vi "testParseCommentsTrailingSlashSlash.vi"(8 "error in (no error)":errorcluster, 11 "testStateMachineUtilities in":refnum<class "testStateMachineUtilities.lvclass">) -> (0 "error out":errorcluster, 3 "testStateMachineUtilities out":refnum<class "testStateMachineUtilities.lvclass">)   [LabVIEW 2020, in "testStateMachineUtilities.lvclass"]
uses:
  testStateMachineUtilities.lvclass
  <userlib>/_OpenG.lib/error/error.llb/openg_error.lvlib
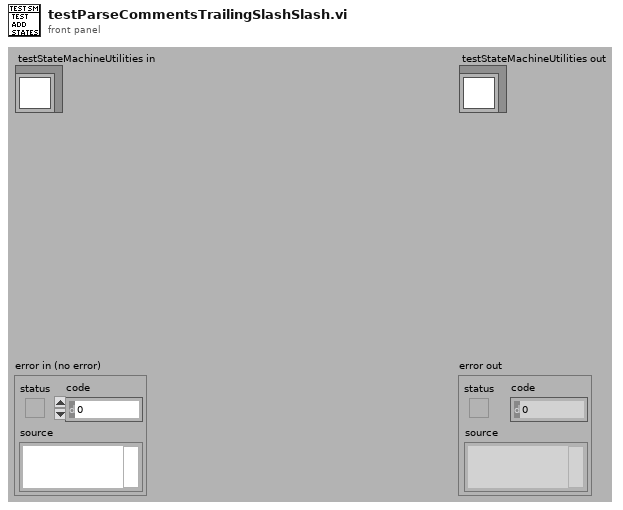
[diagram p1: front panel]
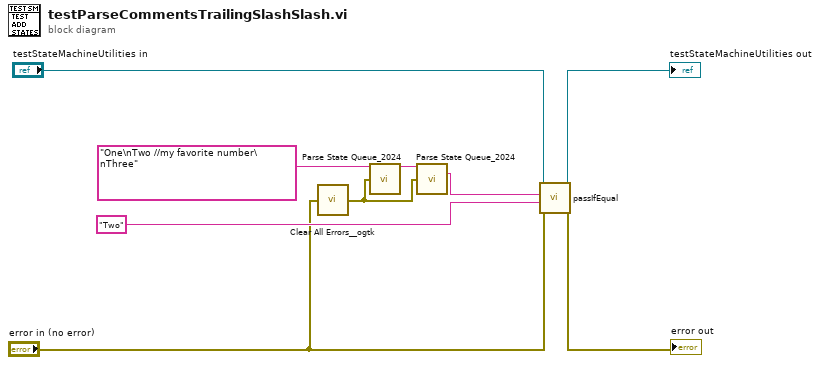
[diagram p0: block diagram]
diagram:
  n1 = call <userlib>:"Clear All Errors__ogtk.vi"("Error In"="error in (no error)") -> ("Error Out"=w1:errorcluster)  [unwired: 3 in]
  n2 = call "Parse State Queue_2024.vi"("State Queue"="One\nTwo //my favorite number\nThree", "Error In (no error)"=w1) -> ("Remaining States"=w5:string)  [unwired: 11 in, 2 out]
  n3 = call "Parse State Queue_2024.vi"("State Queue"=w5, "Error In (no error)"=w1) -> ("Current State"=w4:string)  [unwired: 11 in, 2 out]
  n4 = call-dynamic "passIfEqual.vi"("error in (no error)"="error in (no error)", "y"="Two" ("State Queue"), "x"=w4, "TestCase in"="testStateMachineUtilities in") -> ("error out"=→"error out":errorcluster, "TestCase out"=→"testStateMachineUtilities out":refnum<class "testStateMachineUtilities.lvclass">)  [unwired: 6 in]
